vi "Untitled 1 (SubVI).vi"(11 "Array in":refnum<class "UI_DAQ_config.lvclass">[](array[class])) -> (3 "Array out":refnum<class "UI_DAQ_config.lvclass">[](array[class]))   [LabVIEW 2016]
uses:
  UI_DAQ_config/UI_DAQ_config.lvclass
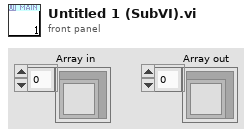
[diagram p1: front panel]
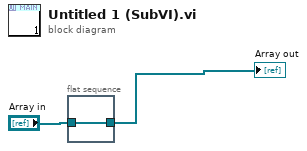
[diagram p0: block diagram]
diagram:
  n1 = flat-sequence {
    tunnel: "Array in" -> [w3]
    tunnel: [w3] -> w2
    frame #0 {
    }
  }
  "Array out" <- w2
